vi "SubVI Tester.vi"() -> ()   [LabVIEW 2015]
uses:
  Control 2.ctl
panel:
  out "weather data out":T1={"Current Temperature"=0.0, "Max Temperature"=0.0, "Min Temperature"=0.0, "Warning Text"="No Warning", "Warning?"=FALSE}
  in  "Min Temperature":dbl=10.0
  in  "Max Temperature":dbl=30.0
  in  "Stop":bool
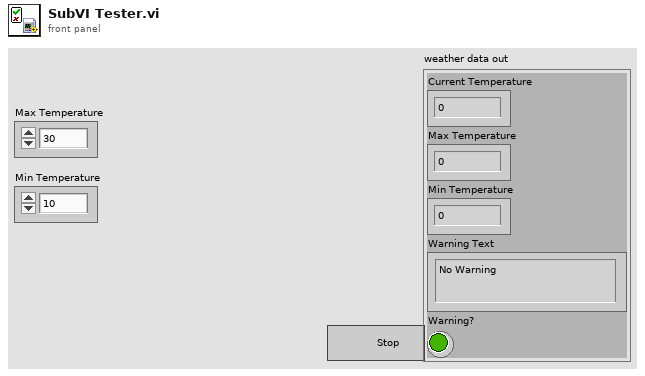
[diagram p1: front panel]
types:
  T1 = cluster{"Current Temperature":dbl, "Max Temperature":dbl, "Min Temperature":dbl, "Warning Text":string, "Warning?":bool}
  T2 = typedef "Control 2.ctl" = cluster{"Current Temperature":dbl, "Max Temperature":dbl, "Min Temperature":dbl, "Warning Text":string, "Warning?":bool}
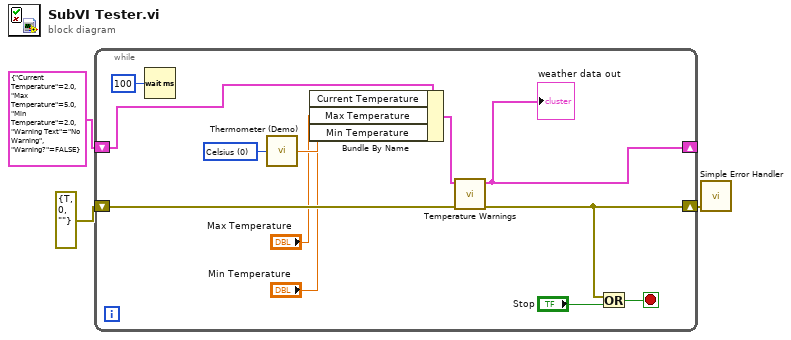
[diagram p0: block diagram]
diagram:
  n1 = while {
    shift-right: [w11] -> w3
    shift-left: errorcluster {"status"=TRUE, "code"=0, "source"=""} ("error out") -> [w12]
    shift-right: [w6] -> _
    shift-left: T2 {"Current Temperature"=2.0, "Max Temperature"=5.0, "Min Temperature"=2.0, "Warning Text"="No Warning", "Warning?"=FALSE} ("weather data in") -> [w4]
    stop <- w13 stop-if-true
    w10 = u16 0 items=["Celsius", "Fahrenheit"] ("Units (0: Celsius)")
    n2 = Wait (ms)(milliseconds to wait=u32 100) -> ()  [unwired: 1 out]
    n3 = call "Thermometer (Demo).vi"("Units (0: Celsius)"=w10) -> ("Temperature Value"=w9:dbl)
    n4 = Bundle By Name(cluster=w4, "Current Temperature"=w9, "Max Temperature"="Max Temperature", "Min Temperature"="Min Temperature") -> (w5:T2)
    n5 = call "Temperature Warnings.vi"("Error In"=w12, "weather data in"=w5) -> ("Error Out"=w11:errorcluster, "weather data out"=w6:T1)  [unwired: 8 in]
    "weather data out" <- w6
    n6 = Or(x=w11, y="Stop") -> (x .or. y?=w13:bool)
  }
  n7 = call <vilib>:"Simple Error Handler.vi"("error in (no error)"=w3) -> ()  [unwired: 4 in, 5 out]
